vi "CreateScanFile.vi"(1 "Meas":T1={"S11"=TRUE, "S12"=TRUE, "S21"=TRUE, "S22"=TRUE}, 2 "Scans":T4(array[cluster]) {"Stop" format="%.9f"; "Start" format="%.9f"}, 3 "PathIn":path) -> (0 "PathOut":path)   [LabVIEW 2017]
uses:
  ScanTarget.ctl
  ScanPara.ctl
  <vilib>/Utility/file.llb/Write Delimited Spreadsheet (string).vi
  <vilib>/Utility/file.llb/Write Delimited Spreadsheet (DBL).vi
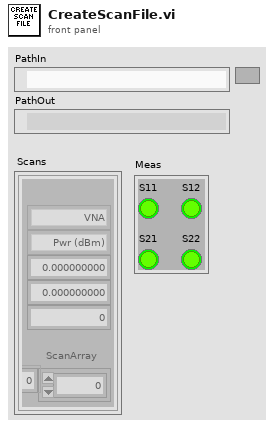
[diagram p1: front panel]
types:
  T1 = cluster{"S11":bool, "S12":bool, "S21":bool, "S22":bool}
  T2 = typedef "ScanTarget.ctl" = enum16{"VNA", "Refrigerator"}
  T3 = typedef "ScanPara.ctl" = enum16{"Freq (GHz)", "Pwr (dBm)", "Temp (K)", "N.A."}
  T4 = cluster{"Target":T2, "Parameter":T3, "Start":dbl, "Stop":dbl, "#Steps":u32, "ScanArray":dbl[]}[]
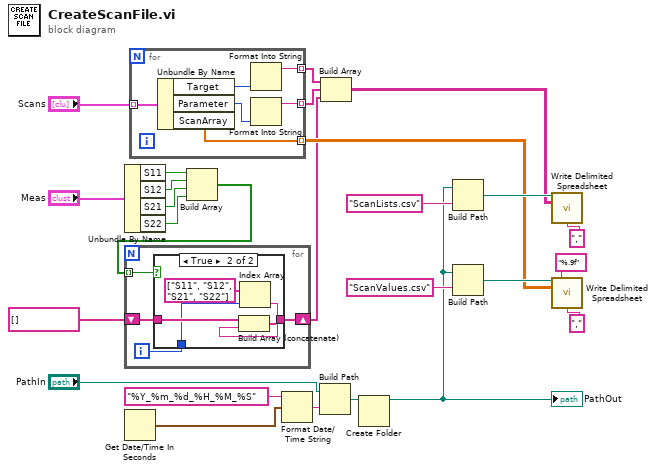
[diagram p0: block diagram]
diagram:
  n1 = Unbundle By Name("Meas") -> ("S11"=w14:bool, "S12"=w13:bool, "S21"=w12:bool, "S22"=w11:bool)
  n2 = Get Date/Time In Seconds() -> (seconds since 1Jan1904=w6:timestamp)
  n3 = for {
    tunnel: "Scans" -> [w32] mode=indexing
    tunnel: [w29] -> w17 mode=indexing
    tunnel: [w28] -> w19 mode=indexing
    tunnel: [w27] -> w18 mode=indexing
    n4 = Unbundle By Name(w32) -> ("Target"=w31:T2, "Parameter"=w30:T3, "ScanArray"=w29:dbl[])
    n5 = Format Into String(w31) -> (resulting string=w28:string)  [unwired: 3 in, 1 out]
    n6 = Format Into String(w30) -> (resulting string=w27:string)  [unwired: 3 in, 1 out]
  }
  n7 = Build Array(w14, w13, w12, w11) -> (w9:bool[])
  n8 = for {
    tunnel: w9 -> [w36] mode=indexing
    shift-right: [w33] -> w7
    shift-left: string[] [] ("appended array") -> [w35]
    i -> [w34]
    n9 = case shown="True" w36 {
      tunnel: w35 -> [w37 w40]
      tunnel: w34 -> [_ w39]
      tunnel: [w37 w38] -> w33
      frame False {
      }
      frame True {
        n10 = Index Array(array=string[] ["S11", "S12", "S21", "S22"] ("appended array"), index=w39) -> (element=w41:string)
        n11 = Build Array (concatenate)(w40, w41) -> (w38:string[])
      }
    }
  }
  n12 = Format Date/Time String(time format string (%c)="%Y_%m_%d_%H_%M_%S", seconds (now)=w6) -> (date/time string=w4:string)  [unwired: 1 in]
  n13 = Build Path(base path="PathIn", name or relative path=w4) -> (appended path=w3:path)
  n14 = Build Array(w19, w18, w7) -> (w16:string[][])
  n15 = Create Folder(path (use dialog)=w3) -> (created path=w1:path)  [unwired: 2 in, 2 out]
  "PathOut" <- w1
  n16 = Build Path(base path=w1, name or relative path="ScanLists.csv") -> (appended path=w23:path)
  n17 = Build Path(base path=w1, name or relative path="ScanValues.csv") -> (appended path=w26:path)
  n18 = call-poly <vilib>:"Write Delimited Spreadsheet.vi"("file path (dialog if empty)"=w23, "2D data"=w16, "delimiter (\\t)"="," ("delimiter (\\t)")) -> ()  [unwired: 11 in, 2 out]
  n19 = call-poly <vilib>:"Write Delimited Spreadsheet.vi"("file path (dialog if empty)"=w26, "format (%.3f)"="%.9f", "2D data"=w17, "delimiter (\\t)"="," ("delimiter (\\t)")) -> ()  [unwired: 10 in, 2 out]
